vi "Get DLL Path.vi"() -> (1 "LG Hub SDK DLL":path)   [LabVIEW 2025, in "Logitech Devices.lvlib"]
uses:
  Logitech Devices.lvlib
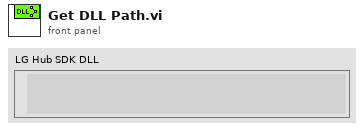
[diagram p1: front panel]
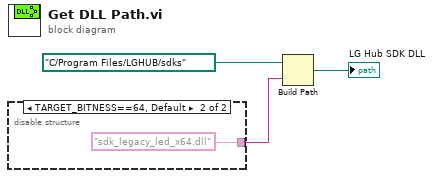
[diagram p0: block diagram]
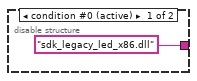
[diagram p2: hidden frame]
diagram:
  n1 = disable-structure shown="TARGET_BITNESS==64, Default" {
    disable-tunnel: ["sdk_legacy_led_x86.dll" "sdk_legacy_led_x64.dll"] -> w1
    frame condition #0 (active) {
    }
    frame condition #1 {
    }
  }
  n2 = Build Path(base path=path "C:/Program Files/LGHUB/sdks" ("LG Hub SDK DLL"), name or relative path=w1) -> (appended path=→"LG Hub SDK DLL":path)
